vi "Asynchronous - Display Debug Information.vi"(8 "Reset Method Timeout?":bool, 11 "Message":string="TRIGGER, reset timeout? ") -> ()   [LabVIEW 2019, in "Ballard Arinc-429 Engine.lvlib"]
uses:
  Ballard Arinc-429 Engine.lvlib
  <vilib>/NI VeriStand/Custom Device Tools/Custom Device Utility Library/Custom Device Utility Library.lvlib
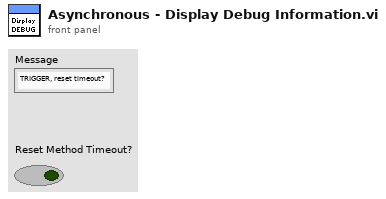
[diagram p1: front panel]
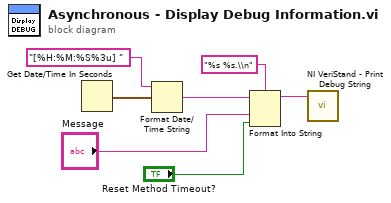
[diagram p0: block diagram]
diagram:
  n1 = Get Date/Time In Seconds() -> (seconds since 1Jan1904=w7:timestamp)
  n2 = Format Date/Time String(time format string (%c)="[%H:%M:%S%3u] ", seconds (now)=w7) -> (date/time string=w5:string)  [unwired: 1 in]
  n3 = Format Into String(format string="%s %s.\\n", initial string=w5, "Message", "Reset Method Timeout?") -> (resulting string=w1:string)  [unwired: 1 in, 1 out]
  n4 = call <vilib>:"NI VeriStand - Print Debug String.vi"("Message"=w1) -> ()  [unwired: 10 in, 1 out]
